vi "Actor Core.vi"(8 "error in":errorcluster, 11 "Controller in":refnum<class "Controller.lvclass">) -> (0 "error out":errorcluster, 3 "Actor out":refnum<class "Actor.lvclass">)   [LabVIEW 2022 SP3, in "Controller.lvlib" / "Controller.lvclass"]
doc: "(<B>Filename</B>: Actor Framework.lvlib:Actor.lvclass:Actor Core.vi)\n\nReceives messages to the actor, reacts to them, and initiates any error handling that may shut the actor down.\n\nDescendant classes may override this VI to append parallel tasks for the actor to complete while it handles messages. Overrides use the Call Parent Class Method node."
uses:
  Controller.lvclass
  <vilib>/ActorFramework/Actor/Actor.lvclass
  Controller.lvclass/Controller.ctl
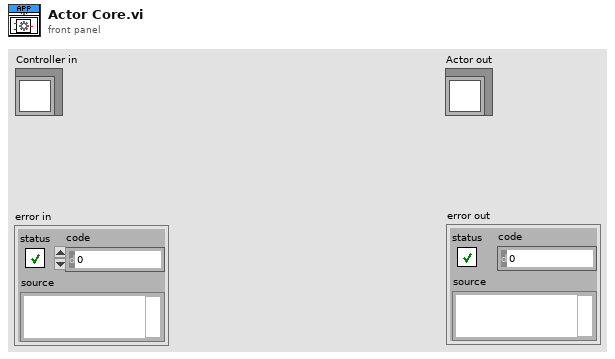
[diagram p1: front panel]
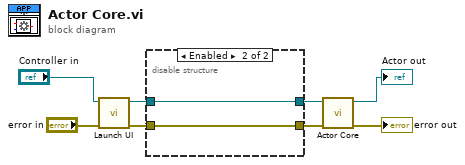
[diagram p0: block diagram]
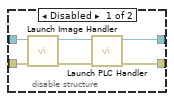
[diagram p2: hidden frame]
diagram:
  n1 = call "Launch UI.vi"("error in (no error)"="error in", "Controller in"="Controller in") -> ("error out"=w1:errorcluster, "Controller out"=w3:refnum<class "Controller.lvclass">)  [unwired: 8 in]
  n2 = disable-structure shown="Enabled" {
    disable-tunnel: [w12 w15] -> w6
    disable-tunnel: [w11 w16] -> w5
    disable-tunnel: w3 -> [w10 w16]
    disable-tunnel: w1 -> [w9 w15]
    frame Disabled {
      n3 = call "Launch Image Handler.vi"("error in (no error)"=w9, "Controller in"=w10) -> ("error out"=w13:errorcluster, "Controller out"=w14:refnum<class "Controller.lvclass">)  [unwired: 8 in]
      n4 = call "Launch PLC Handler.vi"("error in (no error)"=w13, "Controller in"=w14) -> ("error out"=w12:errorcluster, "Controller out"=w11:refnum<class "Controller.lvclass">)  [unwired: 8 in]
    }
    frame Enabled {
    }
  }
  n5 = call-parent "Actor Core.vi"("error in"=w6, "Actor in"=w5) -> ("error out"=→"error out":errorcluster, "Actor out"=→"Actor out":refnum<class "Actor.lvclass">)  [unwired: 8 in]
